vi "Open Playback Files Cropping.vi"(8 "error in (no error)":errorcluster, 11 "Frame Grabber Data In":T1={"Camera Session"="", "Frame"=refnum, "AVI Refnum"=refnum, "Codecs"=[], "Frame number"=0, "Tracking File Refnum"=refnum, "Tick Count"=0, "Probe Object"=refnum, "Playback Probe Data"=[], "Rigid Body"={"Position"={"x (mm)"=0.0, "y (mm)"=0.0, "z (mm)"=0.0}, "Orientation"={"Pitch (rad)"=0.0, "Yaw (rad)"=0.0, "Roll (rad)"=0.0}, "Quaternion"={"qx"=0.0, "qy"=0.0, "qz"=0.0, "qw"=0.0}, "Tracked?"=FALSE}, "Total no frames playback"=0, "Video FPS"=0.0, "Camera connected?"=FALSE, "Scene"=refnum, "Cropped Frame"=refnum, "Tracker FPS"=0.0, "Crop ROI"=[], "Presentation Values"=[], "Elapsed time (ms)"=0, "Camera frames playback"=0, "Refnums"={"Live Refnum"=refnum, "Record Refnum"=refnum, "Recording Settings Refnum"=refnum, "Playback Refnum"=refnum, "Frame Slider Refnum"=refnum, "Pause Refnum"=refnum, "Home Refnum"=refnum, "Crop Refnum"=refnum, "Clear Crop Refnum"=refnum, "stop refnum"=refnum, "Playback Rate Refnum"=refnum, "Operator Settings Refnums"=refnum, "Presentation Refnum"=refnum, "Gestation Refnum"=refnum, "Connection Settings Refnum"=refnum, "Crop Time Frame Slider Refnum"=refnum}, "Dimensions"={"Probe Dimensions"={"Probe Width"=0.0, "Probe Depth"=1.0, "Probe Height"=0.0}, "Room Dimensions"={"Room Width"=0.0, "Room Depth"=0.0, "Room Height"=0.0}}, "Playback Data As Strings"=[], "Cropped Tracking File Refnum"=refnum, "Cropped AVI Refnum"=refnum, "Header"=[]}) -> (0 "error out":errorcluster, 1 "Playback Video":path, 2 "both exist and open?":bool, 3 "Frame Grabber Data Out":T1={"Camera Session"="", "Frame"=refnum, "AVI Refnum"=refnum, "Codecs"=[], "Frame number"=0, "Tracking File Refnum"=refnum, "Tick Count"=0, "Probe Object"=refnum, "Playback Probe Data"=[], "Rigid Body"={"Position"={"x (mm)"=0.0, "y (mm)"=0.0, "z (mm)"=0.0}, "Orientation"={"Pitch (rad)"=0.0, "Yaw (rad)"=0.0, "Roll (rad)"=0.0}, "Quaternion"={"qx"=0.0, "qy"=0.0, "qz"=0.0, "qw"=0.0}, "Tracked?"=FALSE}, "Total no frames playback"=0, "Video FPS"=0.0, "Camera connected?"=FALSE, "Scene"=refnum, "Cropped Frame"=refnum, "Tracker FPS"=0.0, "Crop ROI"=[], "Presentation Values"=[], "Elapsed time (ms)"=0, "Camera frames playback"=0, "Refnums"={"Live Refnum"=refnum, "Record Refnum"=refnum, "Recording Settings Refnum"=refnum, "Playback Refnum"=refnum, "Frame Slider Refnum"=refnum, "Pause Refnum"=refnum, "Home Refnum"=refnum, "Crop Refnum"=refnum, "Clear Crop Refnum"=refnum, "stop refnum"=refnum, "Playback Rate Refnum"=refnum, "Operator Settings Refnums"=refnum, "Presentation Refnum"=refnum, "Gestation Refnum"=refnum, "Connection Settings Refnum"=refnum, "Crop Time Frame Slider Refnum"=refnum}, "Dimensions"={"Probe Dimensions"={"Probe Width"=0.0, "Probe Depth"=1.0, "Probe Height"=0.0}, "Room Dimensions"={"Room Width"=0.0, "Room Depth"=0.0, "Room Height"=0.0}}, "Playback Data As Strings"=[], "Cropped Tracking File Refnum"=refnum, "Cropped AVI Refnum"=refnum, "Header"=[]}, 5 "Number of Playback Frames":i32, 7 "Number of Camera Frames":u32)   [LabVIEW 2017]
uses:
  Controls/Frame Grabber Data.ctl
  <vilib>/userdefined/High Color/IMAQdx.ctl
  <vilib>/vision/Image Controls.llb/IMAQ Image.ctl
  <vilib>/vision/Avi.llb/IMAQ AVI2 Refnum.ctl
  Controls/Rigid Body Info.ctl
  Controls/Position.ctl
  Controls/Orientation.ctl
  Controls/Refnums.ctl
  Controls/Recording Settings.ctl
  Controls/Operator Settings.ctl
  Controls/Operator.ctl
  Controls/Dimensions.ctl
  Controls/Room Dimensions.ctl
  <vilib>/Utility/file.llb/Read Delimited Spreadsheet (string).vi
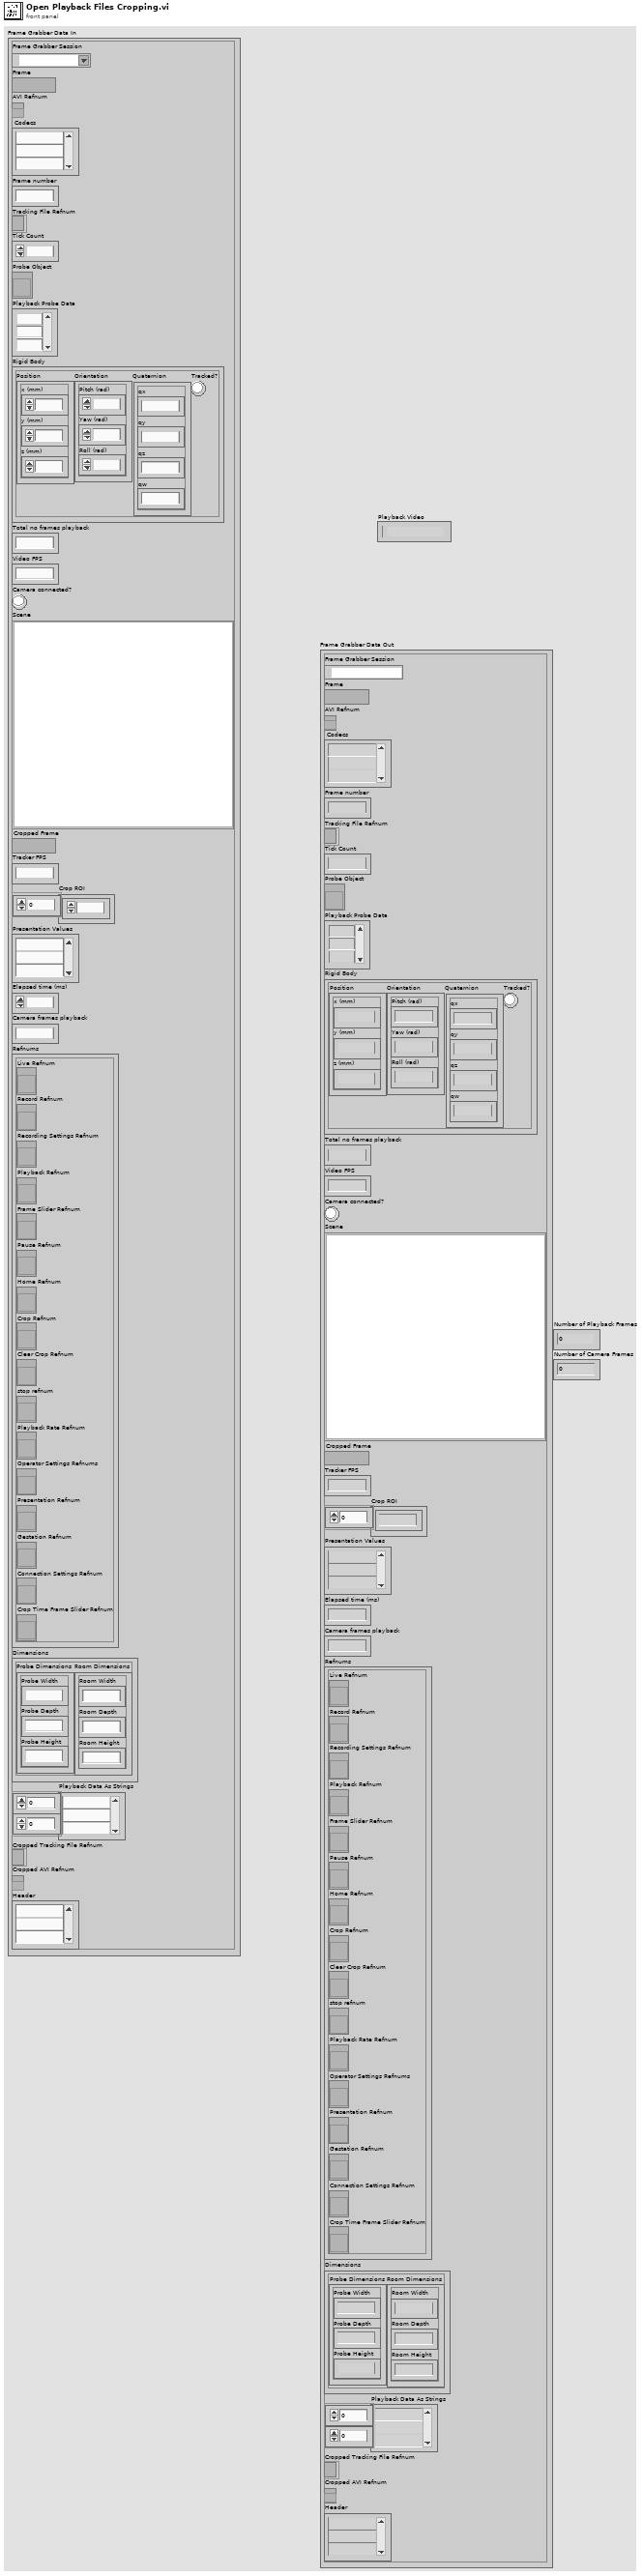
[diagram p1: front panel]
types:
  T1 = typedef "Frame Grabber Data.ctl" = cluster{"Camera Session":T2, "Frame":T3, "AVI Refnum":T4, "Codecs":string[], "Frame number":u32, "Tracking File Refnum":refnum<file>, "Tick Count":u32, "Probe Object":refnum<vi>, "Playback Probe Data":dbl[][], "Rigid Body":T5, "Total no frames playback":i32, "Video FPS":dbl, "Camera connected?":bool, "Scene":refnum<vi>, "Cropped Frame":T3, "Tracker FPS":dbl, "Crop ROI":i32[], "Presentation Values":string[], "Elapsed time (ms)":u32, "Camera frames playback":u32, "Refnums":T8, "Dimensions":T9, "Playback Data As Strings":string[][], "Cropped Tracking File Refnum":refnum<file>, "Cropped AVI Refnum":T4, "Header":string[]}
  T2 = typedef "IMAQdx.ctl" = refnum<k21>
  T3 = typedef "IMAQ Image.ctl" = refnum<image>
  T4 = typedef "IMAQ AVI2 Refnum.ctl" = refnum<k20>
  T5 = typedef "Rigid Body Info.ctl" = cluster{"Position":T6, "Orientation":T7, "Quaternion":cluster{"qx":sgl, "qy":sgl, "qz":sgl, "qw":sgl}, "Tracked?":bool}
  T6 = typedef "Position.ctl" = cluster{"x (mm)":sgl, "y (mm)":sgl, "z (mm)":sgl}
  T7 = typedef "Orientation.ctl" = cluster{"Pitch (rad)":sgl, "Yaw (rad)":sgl, "Roll (rad)":sgl}
  T8 = typedef "Refnums.ctl" = cluster{"Live Refnum":refnum<vi>, "Record Refnum":refnum<vi>, "Recording Settings Refnum":refnum<vi>, "Playback Refnum":refnum<vi>, "Frame Slider Refnum":refnum<vi>, "Pause Refnum":refnum<vi>, "Home Refnum":refnum<vi>, "Crop Refnum":refnum<vi>, "Clear Crop Refnum":refnum<vi>, "stop refnum":refnum<vi>, "Playback Rate Refnum":refnum<vi>, "Operator Settings Refnums":refnum<vi>, "Presentation Refnum":refnum<vi>, "Gestation Refnum":refnum<vi>, "Connection Settings Refnum":refnum<vi>, "Crop Time Frame Slider Refnum":refnum<vi>}
  T9 = typedef "Dimensions.ctl" = cluster{"Probe Dimensions":cluster{"Probe Width":sgl, "Probe Depth":sgl, "Probe Height":sgl}, "Room Dimensions":T10}
  T10 = typedef "Room Dimensions.ctl" = cluster{"Room Width":dbl, "Room Depth":dbl, "Room Height":dbl}
  T11 = enum16{"open", "replace", "create", "open or create", "replace or create", "replace or create with confirmation"}
  T12 = cluster{"Width":u32, "Height":u32, "Frames Per Second":u32, "Codec":string, "Has Data":bool}
  T13 = cluster{"Scale.Range:Minimum":i32, "Number of Frames":i32, "Scale.Range:Minimum":i32}
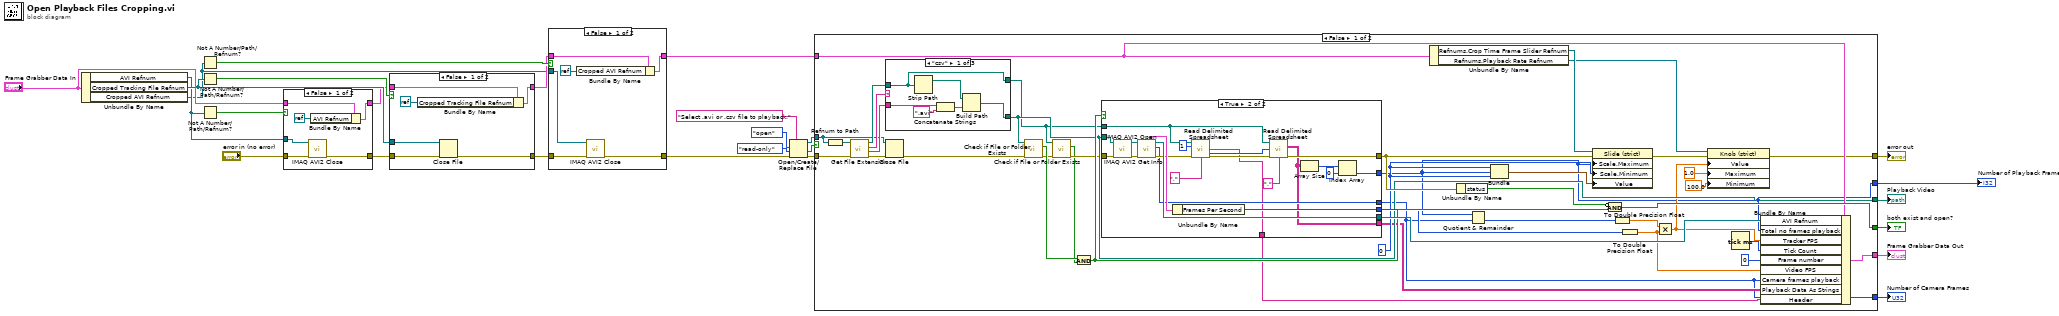
[diagram p0: block diagram]
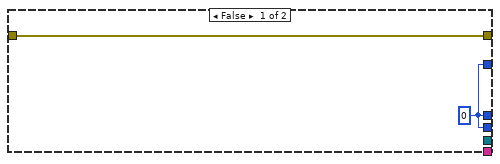
[diagram p5: hidden frame]
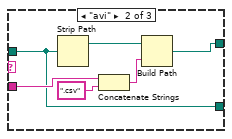
[diagram p6: hidden frame]
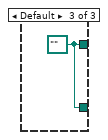
[diagram p7: hidden frame]
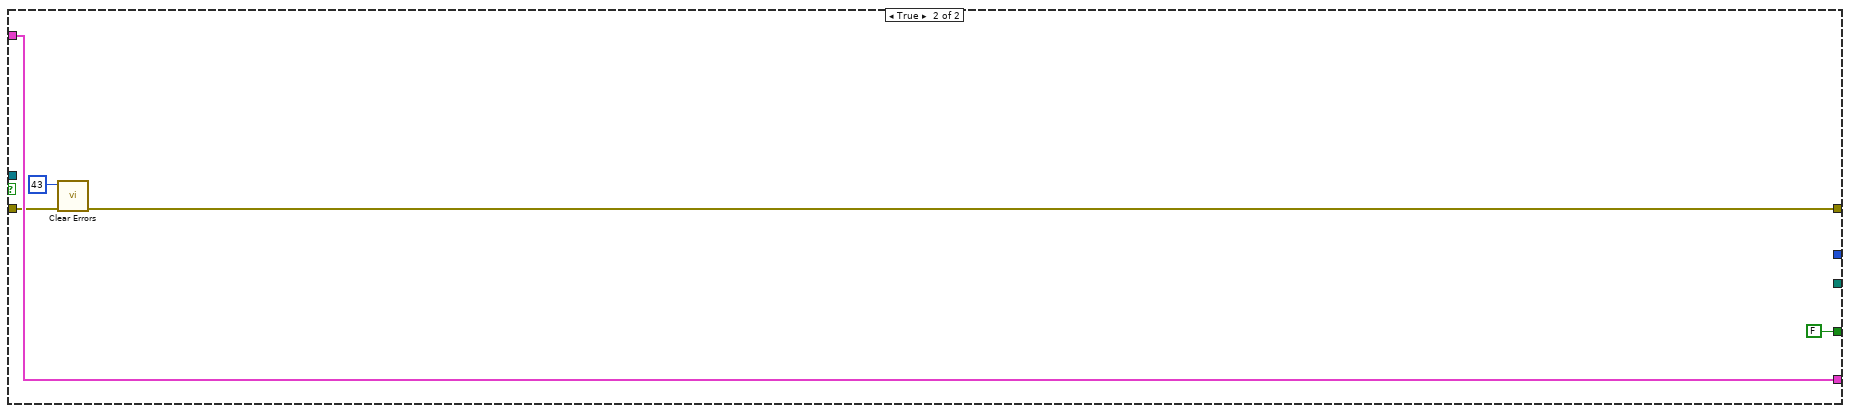
[diagram p8: hidden frame]
diagram:
  n1 = Unbundle By Name("Frame Grabber Data In") -> ("AVI Refnum"=w7:T4, "Cropped Tracking File Refnum"=w8:refnum<file>, "Cropped AVI Refnum"=w3:T4)
  n2 = Not A Number/Path/Refnum?(number/path/refnum=w3) -> (NaN/Path/Refnum?=w14:bool)
  n3 = Not A Number/Path/Refnum?(number/path/refnum=w8) -> (NaN/Path/Refnum?=w15:bool)
  n4 = Not A Number/Path/Refnum?(number/path/refnum=w7) -> (NaN/Path/Refnum?=w12:bool)
  n5 = case shown="False" w12 {
    tunnel: "error in (no error)" -> [w32 w34]
    tunnel: [w31 w34] -> w10
    tunnel: "Frame Grabber Data In" -> [w30 w33]
    tunnel: w7 -> [w29 _]
    tunnel: [w28 w33] -> w6
    frame False {
      n6 = call "IMAQ AVI2 Close"("error in (no error)"=w32, "AVI Refnum"=w29) -> ("error out"=w31:errorcluster)  [unwired: 9 in]
      n7 = Bundle By Name(cluster=w30, "AVI Refnum"=refnum<k0> refnum) -> (w28:T1)
    }
    frame True {
    }
  }
  n8 = case shown="False" w15 {
    tunnel: w10 -> [w40 w42]
    tunnel: [w39 w42] -> w16
    tunnel: w6 -> [w38 w41]
    tunnel: w8 -> [w37 _]
    tunnel: [w35 w41] -> w5
    frame False {
      n9 = Bundle By Name(cluster=w38, "Cropped Tracking File Refnum"=refnum<k0> refnum) -> (w35:T1)
      n10 = Close File(refnum=w37, error in=w40) -> (error out=w39:errorcluster)  [unwired: 1 out]
    }
    frame True {
    }
  }
  n11 = case shown="False" w14 {
    tunnel: w16 -> [w48 w50]
    tunnel: [w47 w50] -> w13
    tunnel: w5 -> [w46 w49]
    tunnel: [w45 w49] -> w4
    tunnel: w3 -> [w43 _]
    frame False {
      n12 = Bundle By Name(cluster=w46, "Cropped AVI Refnum"=refnum<k0> refnum) -> (w45:T1)
      n13 = call "IMAQ AVI2 Close"("error in (no error)"=w48, "AVI Refnum"=w43) -> ("error out"=w47:errorcluster)  [unwired: 9 in]
    }
    frame True {
    }
  }
  n14 = Open/Create/Replace File(error in=w13, prompt="Select .avi or .csv file to playback.", operation (0:open)=T11."open", access (0:read/write)=enum16{"read/write", "read-only", "write-only"}."read-only") -> (refnum out=w25:refnum<file>, cancelled=w19:bool, error out=w26:errorcluster)  [unwired: 2 in]
  n15 = case shown="False" w19 {
    tunnel: w26 -> [w90 w129]
    tunnel: w25 -> [w73 _]
    tunnel: w4 -> [w78 w131]
    tunnel: [w83 FALSE] -> w21
    tunnel: [w81 w131] -> w20
    tunnel: [w71 _] -> w18
    tunnel: [w58 w127] -> w17
    tunnel: [w53 _] -> w2
    tunnel: [w52 _] -> w1
    frame False {
      w56 = 0 ("Scale.Range:Minimum")
      n16 = Refnum to Path(1:w73) -> (0:w89:path)
      n17 = call <vilib>:"Get File Extension.vi"("error in (no error)"=w90, "file"=w89) -> ("error out"=w74:errorcluster, "filename without extension"=w87:string, "lowercase file extension"=w88:string, "dup file"=w86:path)  [unwired: 5 in, 1 out]
      n18 = case shown="\"csv\"" w88 {
        tunnel: w87 -> [w119 w124 _]
        tunnel: w86 -> [w116 w123 _]
        tunnel: [w114 w123 w126] -> w71
        tunnel: [w116 w120 w126] -> w68
        frame "csv" {
          n19 = Strip Path(path=w116) -> (stripped path=w117:path)  [unwired: 1 out]
          n20 = Concatenate Strings(w119, ".avi" ("string")) -> (w115:string)
          n21 = Build Path(base path=w117, name or relative path=w115) -> (appended path=w114:path)
        }
        frame "avi" {
          n22 = Strip Path(path=w123) -> (stripped path=w122:path)  [unwired: 1 out]
          n23 = Concatenate Strings(w124, ".csv" ("string")) -> (w121:string)
          n24 = Build Path(base path=w122, name or relative path=w121) -> (appended path=w120:path)
        }
        frame Default {
          w126 = path "" ("dup file")
        }
      }
      n25 = Close File(refnum=w73, error in=w74) -> (error out=w72:errorcluster)  [unwired: 1 out]
      n26 = call <vilib>:"Check if File or Folder Exists.vi"("error in (no error)"=w72, "path"=w71) -> ("error out"=w66:errorcluster, "file or folder exists?"=w70:bool)  [unwired: 7 in, 1 out]
      n27 = call <vilib>:"Check if File or Folder Exists.vi"("error in (no error)"=w66, "path"=w68) -> ("error out"=w69:errorcluster, "file or folder exists?"=w67:bool)  [unwired: 7 in, 1 out]
      n28 = And(x=w70, y=w67) -> (x .and. y?=w84:bool)
      n29 = case shown="True" w84 {
        tunnel: w69 -> [w92 w107]
        tunnel: w71 -> [_ w113]
        tunnel: [w92 w100] -> w79
        tunnel: [_ w110] -> w85
        tunnel: w68 -> [_ w103]
        tunnel: [w91 w104] -> w52
        tunnel: [w91 w108] -> w75
        tunnel: [w91 w98] -> w53
        tunnel: [_ w99] -> w55
        tunnel: [_ w94] -> w51
        frame False {
          w91 = 0 ("Number of Frames")
        }
        frame True {
          n30 = call "IMAQ AVI2 Open"("error in (no error)"=w107, "AVI File Path"=w113) -> ("error out"=w112:errorcluster, "AVI Refnum"=w111:T4)  [unwired: 8 in]
          n31 = call "IMAQ AVI2 Get Info"("error in (no error)"=w112, "AVI Refnum"=w111) -> ("error out"=w106:errorcluster, "Number of Frames"=w104:u32, "AVI Refnum (duplicate)"=w110:T4, "Frame Data"=w109:T12)  [unwired: 5 in, 1 out]
          n32 = Unbundle By Name(w109) -> ("Frames Per Second"=w108:u32)
          n33 = call-poly <vilib>:"Read Delimited Spreadsheet.vi"("file path (dialog if empty)"=w103, "number of rows (all:-1)"=1, "error in (no error)"=w106, "delimiter (\\t)"="," ("delimiter (\\t)")) -> ("first row"=w94:string[], "mark after read (chars.)"=w101:i32, "error out"=w102:errorcluster)  [unwired: 6 in, 3 out]
          n34 = call-poly <vilib>:"Read Delimited Spreadsheet.vi"("file path (dialog if empty)"=w103, "start of read offset (chars.:0)"=w101, "error in (no error)"=w102, "delimiter (\\t)"="," ("delimiter (\\t)")) -> ("all rows"=w99:string[][], "error out"=w100:errorcluster)  [unwired: 6 in, 4 out]
          n35 = Array Size(array=w99) -> (size(s)=w97:i32[])
          n36 = Index Array(array=w97, index=0) -> (element=w98:i32)
        }
      }
      n37 = Unbundle By Name(w78) -> ("Refnums.Crop Time Frame Slider Refnum"=w77:refnum<vi>, "Refnums.Playback Rate Refnum"=w65:refnum<vi>)
      n38 = Unbundle By Name(w79) -> ("status"=w82:bool)
      n39 = Quotient & Remainder(x=w53, y=w52) -> (floor(x/y)=w76:u32)  [unwired: 1 out]
      n40 = Bundle("Scale.Range:Minimum"=w56, "Number of Frames"=w53, "Scale.Range:Minimum"=w56) -> (w57:T13)  [unwired: 1 in]
      n41 = property class="Slide (strict)"(reference=w77, error in=w79, "Scale.Maximum"=w53, "Scale.Minimum"=w56, "Value"=w57) -> (error out=w63:errorcluster)  [unwired: 1 out]
      n42 = Compound Arithmetic op=AND(invert w82, w84) -> (w83:bool)
      n43 = To Double Precision Float(number=w76) -> (double precision float=w59:dbl)
      n44 = To Double Precision Float(number=w75) -> (double precision float=w60:dbl)
      n45 = Multiply(x=w59, y=w60) -> (x*y=w64:dbl)
      n46 = property class="Knob (strict)"(reference=w65, error in=w63, "Value"=w64, "Maximum"=1.0 ("Data Entry Limits:Maximum"), "Minimum"=100.0 ("Data Entry Limits:Minimum")) -> (error out=w58:errorcluster)  [unwired: 1 out]
      n47 = Tick Count (ms)() -> (millisecond timer value=w80:u32)
      n48 = Bundle By Name(cluster=w78, "AVI Refnum"=w85, "Total no frames playback"=w53, "Tracker FPS"=w64, "Tick Count"=w80, "Frame number"=u32 0, "Video FPS"=w60, "Camera frames playback"=w52, "Playback Data As Strings"=w55, "Header"=w51) -> (w81:T1)
    }
    frame True {
      n49 = call <vilib>:"Clear Errors.vi"("error in (no error)"=w129, "specific error code to clear (0: all)"=43) -> ("error out"=w127:errorcluster)  [unwired: 4 in, 1 out]
    }
  }
  "both exist and open?" <- w21
  "Frame Grabber Data Out" <- w20
  "Playback Video" <- w18
  "error out" <- w17
  "Number of Playback Frames" <- w2
  "Number of Camera Frames" <- w1
